vi "Parse Video Config File.vi"(4 "error in (no error)":errorcluster, 6 "Config File Path":path) -> (0 "error out":errorcluster, 1 "Streaming Intrinsics":T1, 2 "Color Path":path, 3 "Depth Path":path)   [LabVIEW 2018]
uses:
  Video Intrinsics STYP.ctl
  <vilib>/Utility/config.llb/Read Key (Path).vi
  <vilib>/Utility/config.llb/Read Key (Double).vi
  <vilib>/Utility/config.llb/NI_LVConfig.lvlib
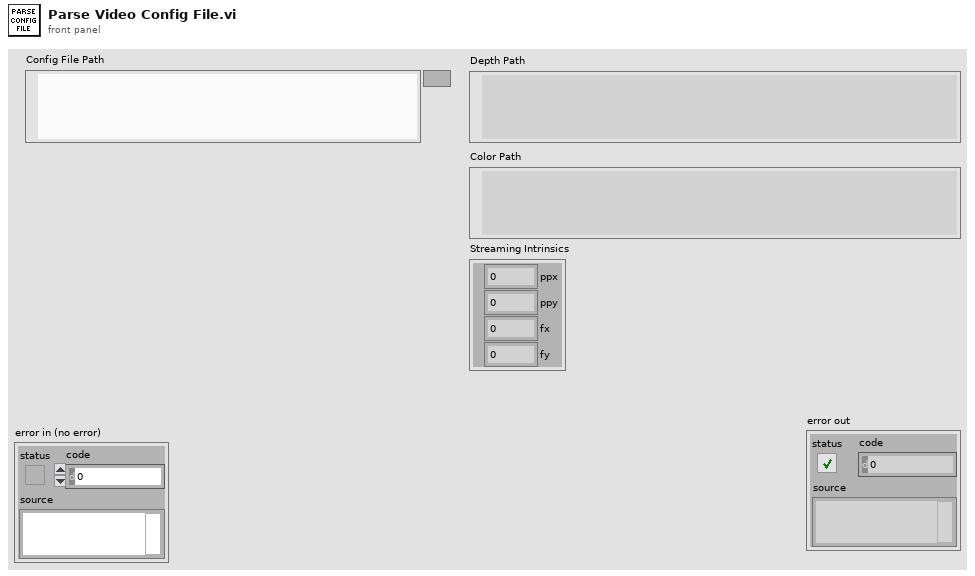
[diagram p1: front panel]
types:
  T1 = typedef "Video Intrinsics STYP.ctl" = cluster{"ppx":sgl, "ppy":sgl, "fx":sgl, "fy":sgl}
  T2 = typedef "NI_LVConfig.lvlib/Config Data RefNum.ctl" = refnum<k1>
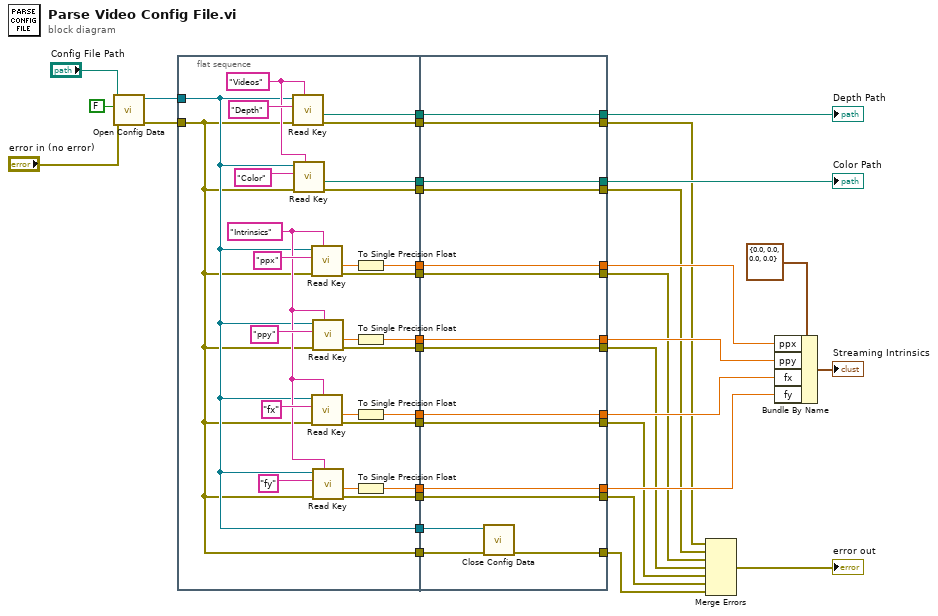
[diagram p0: block diagram]
diagram:
  n1 = call <vilib>:"Open Config Data.vi"("error in (no error)"="error in (no error)", "create file if necessary (T)"=FALSE, "configuration file path"="Config File Path") -> ("error out"=w32:errorcluster, "refnum"=w5:T2)  [unwired: 6 in, 1 out]
  n2 = flat-sequence {
    tunnel: w32 -> [w36]
    tunnel: w5 -> [w37]
    tunnel: [w49] -> w17
    tunnel: [w48] -> w16
    tunnel: [w47] -> w15
    tunnel: [w46] -> w14
    tunnel: [w45] -> w13
    tunnel: [w44] -> w12
    tunnel: [w43] -> w11
    tunnel: [w42] -> w10
    tunnel: [w41] -> w9
    tunnel: [w40] -> w8
    tunnel: [w39] -> w7
    tunnel: [w38] -> w6
    tunnel: [w37] -> w4
    tunnel: [w36] -> w3
    tunnel: [w65] -> w18
    tunnel: [w66] -> w19
    tunnel: [w67] -> w20
    tunnel: [w68] -> w21
    tunnel: [w69] -> w22
    tunnel: [w70] -> w23
    tunnel: [w71] -> w24
    tunnel: [w72] -> w25
    tunnel: [w73] -> w27
    tunnel: [w74] -> w28
    tunnel: [w75] -> w29
    tunnel: [w76] -> w30
    tunnel: w17 -> [w76]
    tunnel: w16 -> [w75]
    tunnel: w15 -> [w74]
    tunnel: w14 -> [w73]
    tunnel: w13 -> [w72]
    tunnel: w12 -> [w71]
    tunnel: w11 -> [w70]
    tunnel: w10 -> [w69]
    tunnel: w9 -> [w68]
    tunnel: w8 -> [w67]
    tunnel: w7 -> [w66]
    tunnel: w6 -> [w65]
    tunnel: w4 -> [w64]
    tunnel: w3 -> [w63]
    tunnel: [w62] -> w2
    frame #0 {
      w54 = "Intrinsics" ("section")
      w60 = "Videos" ("section")
      n3 = call-poly <vilib>:"Read Key.vi"("section"=w60, "error in (no error)"=w36, "key"="Depth", "refnum"=w37) -> ("error out"=w43:errorcluster, "value"=w45:path)  [unwired: 4 in, 2 out]
      n4 = call-poly <vilib>:"Read Key.vi"("section"=w60, "error in (no error)"=w36, "key"="Color", "refnum"=w37) -> ("error out"=w42:errorcluster, "value"=w44:path)  [unwired: 4 in, 2 out]
      n5 = call-poly <vilib>:"Read Key.vi"("section"=w54, "error in (no error)"=w36, "key"="ppx", "refnum"=w37) -> ("error out"=w41:errorcluster, "value"=w53:dbl)  [unwired: 4 in, 2 out]
      n6 = call-poly <vilib>:"Read Key.vi"("section"=w54, "error in (no error)"=w36, "key"="fx", "refnum"=w37) -> ("error out"=w39:errorcluster, "value"=w51:dbl)  [unwired: 4 in, 2 out]
      n7 = call-poly <vilib>:"Read Key.vi"("section"=w54, "error in (no error)"=w36, "key"="ppy", "refnum"=w37) -> ("error out"=w40:errorcluster, "value"=w52:dbl)  [unwired: 4 in, 2 out]
      n8 = call-poly <vilib>:"Read Key.vi"("section"=w54, "error in (no error)"=w36, "key"="fy", "refnum"=w37) -> ("error out"=w38:errorcluster, "value"=w50:dbl)  [unwired: 4 in, 2 out]
      n9 = To Single Precision Float(number=w53) -> (single precision float=w49:sgl)
      n10 = To Single Precision Float(number=w52) -> (single precision float=w48:sgl)
      n11 = To Single Precision Float(number=w51) -> (single precision float=w47:sgl)
      n12 = To Single Precision Float(number=w50) -> (single precision float=w46:sgl)
    }
    frame #1 {
      n13 = call <vilib>:"Close Config Data.vi"("error in (no error)"=w63, "refnum"=w64) -> ("error out"=w62:errorcluster)  [unwired: 8 in, 1 out]
    }
  }
  n14 = Merge Errors(w23, w22, w21, w20, w19, w18, w2) -> (→"error out":errorcluster)
  n15 = Bundle By Name(cluster=T1 {"ppx"=0.0, "ppy"=0.0, "fx"=0.0, "fy"=0.0} ("Streaming Intrinsics 2"), "ppx"=w30, "ppy"=w29, "fx"=w28, "fy"=w27) -> (→"Streaming Intrinsics":T1)
  "Depth Path" <- w25
  "Color Path" <- w24
